vi "AutoAim.vi"(8 "error in (no error)":errorcluster, 10 "InitialCall":bool, 11 "RobotDriveDevRef":T1={"DevStatus"={"status"=FALSE, "code"=0, "source"=""}, "Motors[]"=[], "Square Inputs"=FALSE, "Max Output"=1.0, "Isochronous"=FALSE}) -> (0 "error out":errorcluster, 2 "CleartoLaunch(Gyro)":bool)   [LabVIEW 2013]
uses:
  <vilib>/Rock Robotics/WPI/RobotDrive/WPI_RobotDriveDevRef.ctl
  <vilib>/Rock Robotics/WPI/MotorControl/WPI_MotorControlDeviceRef.ctl
  <vilib>/Rock Robotics/SystemInterfaces/Typedef/FPGA_TypedefDigitalModule.ctl
  <vilib>/Rock Robotics/SystemInterfaces/DIO/FPGA_DIOPWMChannel.ctl
  <vilib>/Rock Robotics/WPI/PWM/WPI_PWMDeadband.ctl
  <vilib>/Rock Robotics/WPI/CAN/Jaguar/SubVIs/WPI_CANJaguar_ControlMode.ctl
  <vilib>/Rock Robotics/WPI/PWM/WPI_PWMTransform_ConPane.ctl
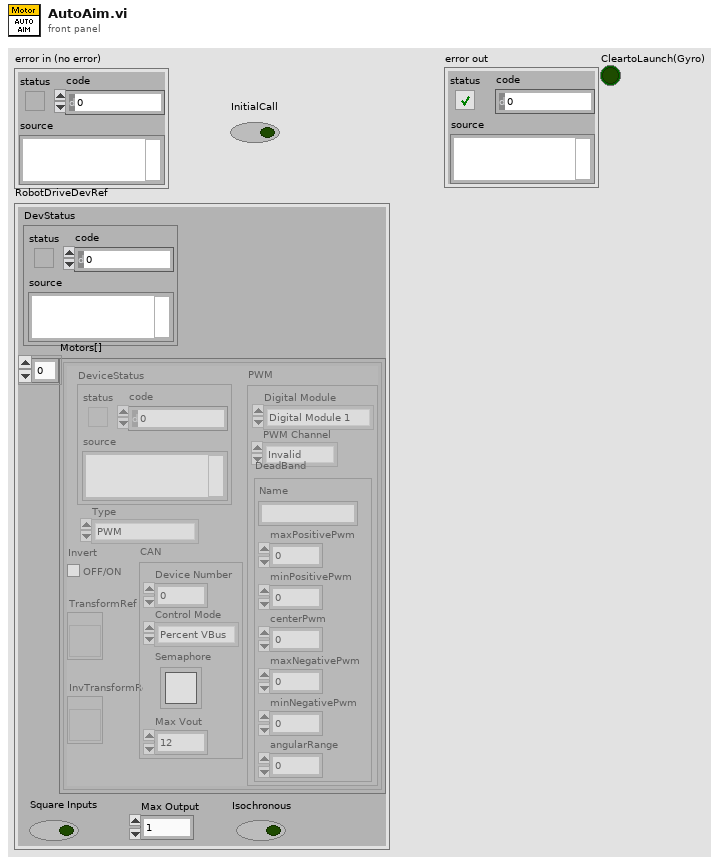
[diagram p1: front panel]
types:
  T1 = typedef "WPI_RobotDriveDevRef.ctl" = cluster{"DevStatus":errorcluster, "Motors[]":T2[], "Square Inputs":bool, "Max Output":dbl, "Isochronous":bool}
  T2 = typedef "WPI_MotorControlDeviceRef.ctl" = cluster{"DeviceStatus":errorcluster, "Type":enum16{"PWM", "CAN"}, "PWM":cluster{"Digital Module":T3, "PWM Channel":T4, "DeadBand":T5}, "CAN":cluster{"Device Number":u8, "Control Mode":T6, "Semaphore":T7, "Max Vout":dbl}, "Invert":bool, "TransformRef":T8, "InvTransformRef":T8}
  T3 = typedef "FPGA_TypedefDigitalModule.ctl" = enum16{"Digital Module 1", "Digital Module 2"}
  T4 = typedef "FPGA_DIOPWMChannel.ctl" = enum8{"PWM 1", "PWM 2", "PWM 3", "PWM 4", "PWM 5", "PWM 6", "PWM 7", "PWM 8", "PWM 9", "PWM 10", "Invalid"}
  T5 = typedef "WPI_PWMDeadband.ctl" = cluster{"Name":string, "maxPositivePwm":i32, "minPositivePwm":i32, "centerPwm":i32, "maxNegativePwm":i32, "minNegativePwm":i32, "angularRange":u16}
  T6 = typedef "WPI_CANJaguar_ControlMode.ctl" = enum8{"Percent VBus", "Current", "Speed", "Position", "Voltage"}
  T7 = typedef "Semaphore RefNum" = refnum<k1>
  T8 = typedef "WPI_PWMTransform_ConPane.ctl" = refnum<vi>
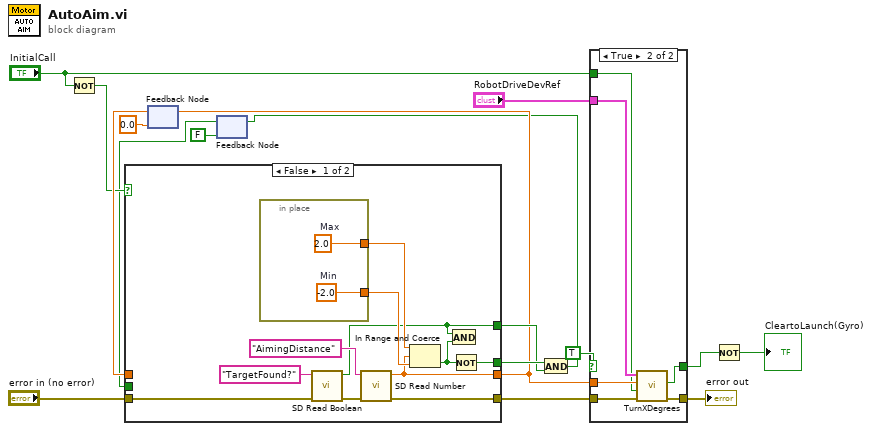
[diagram p0: block diagram]
diagram:
  n1 = Not(x="InitialCall") -> (.not. x?=w9:bool)
  n2 = feedback #1(0.0 ("Numeric")) -> (w13:dbl)
  n3 = feedback #2(FALSE) -> (w4:bool)
  n4 = case shown="False" w9 {
    tunnel: [w23 w31] -> w16
    tunnel: [w22 w33] -> w6
    tunnel: [w21 w31] -> w15
    tunnel: w13 -> [_ w33]
    tunnel: "error in (no error)" -> [w20 w32]
    tunnel: [w18 w32] -> w10
    tunnel: w4 -> [_ w31]
    frame False {
      n5 = in-place {
        in-place-border: [w30] -> w26
        in-place-border: [w29] -> w25
        w29 = -2.0  # Min
        w30 = 2.0  # Max
      }
      n6 = call <vilib>:"SD Read Boolean.vi"("error in"=w20, "Name"="TargetFound?") -> ("error out"=w19:errorcluster, "Boolean"=w21:bool)  [unwired: 7 in, 1 out]
      n7 = call <vilib>:"SD Read Number.vi"("error in"=w19, "Name"="AimingDistance") -> ("error out"=w18:errorcluster, "Numeric"=w22:dbl)  [unwired: 7 in, 1 out]
      n8 = In Range and Coerce(upper limit=w26, x=w22, lower limit=w25) -> (In Range?=w24:bool)  [unwired: 1 out]
      n9 = And(x=w21, y=w24) -> ()  [unwired: 1 out]
      n10 = Not(x=w24) -> (.not. x?=w23:bool)
    }
    frame True {
    }
  }
  n11 = feedback-in #1(w6) -> ()
  n12 = And(x=w16, y=w15) -> (x .and. y?=w2:bool)
  n13 = feedback-in #2(w2) -> ()
  n14 = case shown="True" TRUE {
    selector: TRUE -> [w34 _]
    tunnel: w10 -> [w35 w41]
    tunnel: [w35 w40] -> w17
    tunnel: w6 -> [_ w39]
    tunnel: [w34 w38] -> w8
    tunnel: "RobotDriveDevRef" -> [_ w37]
    tunnel: "InitialCall" -> [_ w36]
    frame False {
    }
    frame True {
      n15 = call "TurnXDegrees.vi"("error in (no error)"=w41, "Reset?"=w36, "degrees"=w39, "RobotDriveDevRef"=w37) -> ("error out"=w40:errorcluster, "Running"=w38:bool)  [unwired: 6 in]
    }
  }
  "error out" <- w17
  n16 = Not(x=w8) -> (.not. x?=→"CleartoLaunch(Gyro)":bool)
